vi "New Mapped Lookup.vi"(8 "error in (no error)":errorcluster) -> (0 "error out":errorcluster, 3 "New Mapped Lookup":refnum<data-value>)   [LabVIEW 2019, in "Lookup API.lvlib" / "Mapped Lookup.lvclass"]
doc: "<b>Description</b> Creates a new Lookup (using the Map Lookup provider).\n\n<b>Outputs</b>\n<b>New Mapped Lookup</b>: A new lookup.\n\nBSD 3-Clause License\n\nCopyright (c) 2021, TauTerra, LLC\nAll rights reserved.\n\nRedistribution and use in source and binary forms, with or without\nmodification, are permitted provided that the following conditions are met:\n\n1. Redistributions of source code must retain the above copyright notice, this\n list of conditions and the following disclaimer.\n\n2. Redistributions in binary form must reproduce the above copyright notice,\n this list of conditions and the following disclaimer in the documentation\n and/or other materials provided with the distribution.\n\n3. Neither the name of the copyright holder nor the names of its\n contributors may be used to endorse or promote products derived from\n this software without specific prior written permission.\n\nTHIS SOFTWARE IS PROVIDED BY THE COPYRIGHT HOLDERS AND CONTRIBUTORS \"AS IS\"\nAND ANY EXPRESS OR IMPLIED WARRANTIES, INCLUDING, BUT NOT LIMITED TO, THE\nIMPLIED WARRANTIES OF MERCHANTABILITY AND FITNESS FOR A PARTICULAR PURPOSE ARE\nDISCLAIMED. IN NO EVENT SHALL THE COPYRIGHT HOLDER OR CONTRIBUTORS BE LIABLE\nFOR ANY DIRECT, INDIRECT, INCIDENTAL, SPECIAL, EXEMPLARY, OR CONSEQUENTIAL\nDAMAGES (INCLUDING, BUT NOT LIMITED TO, PROCUREMENT OF SUBSTITUTE GOODS OR\nSERVICES; LOSS OF USE, DATA, OR PROFITS; OR BUSINESS INTERRUPTION) HOWEVER\nCAUSED AND ON ANY THEORY OF LIABILITY, WHETHER IN CONTRACT, STRICT LIABILITY,\nOR TORT (INCLUDING NEGLIGENCE OR OTHERWISE) ARISING IN ANY WAY OUT OF THE USE\nOF THIS SOFTWARE, EVEN IF ADVISED OF THE POSSIBILITY OF SUCH DAMAGE."
uses:
  Mapped Lookup.lvclass
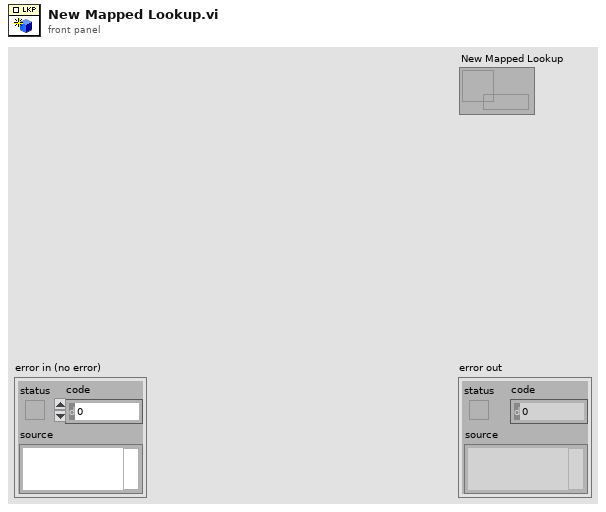
[diagram p1: front panel]
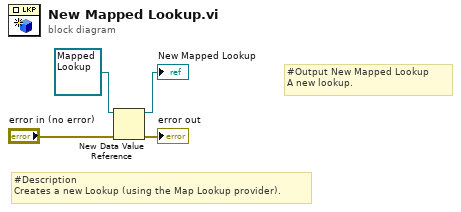
[diagram p0: block diagram]
diagram:
  # "#Output New Mapped Lookup\nA new lookup."
  # "#Description\nCreates a new Lookup (using the Map Lookup provider)."
  n1 = New Data Value Reference(data value=refnum<class "Mapped Lookup.lvclass"> refnum ("Mapped Lookup in"), error in="error in (no error)") -> (data value reference=→"New Mapped Lookup":refnum<data-value>, error out=→"error out":errorcluster)
